vi "测量值存进数据库练习.vi"() -> ()   [LabVIEW 2025]
uses:
  <vilib>/Instr/_visa.llb/VISA Configure Serial Port (Instr).vi
panel:
  out "转换为十进制数据":u32
  out "地址01的光亮度数据":dbl
  out "字符串显示·的十六进制数据":string
  out "无符号字节数组":u8[](array[numeric])
  out "十六进制整形字符串":string[](array[string])
  out "提取的从机地址01的亮度原始数据":string
  out "所有测量记录":string[][](table)
  out "获取下位机返回的原始数据包":string
  in  "发送命令":string
  in  "波特率":u32=9600 caption="波特率(9600)"
  in  "选择串口":refnum<visa-resource-name>
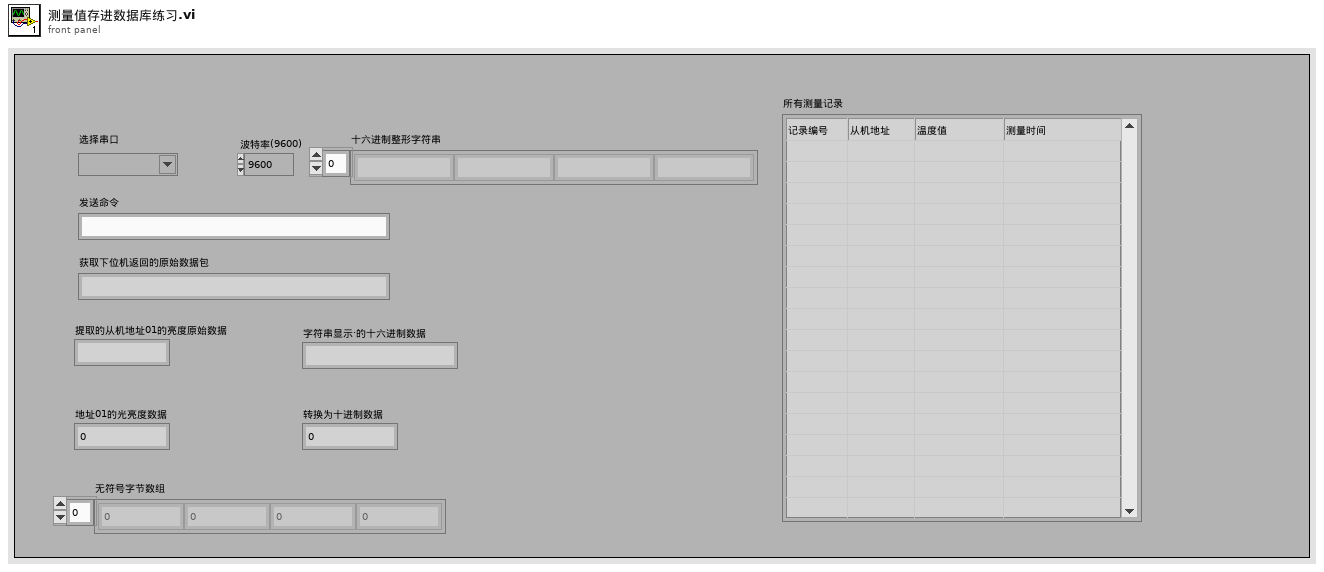
[diagram p1: front panel]
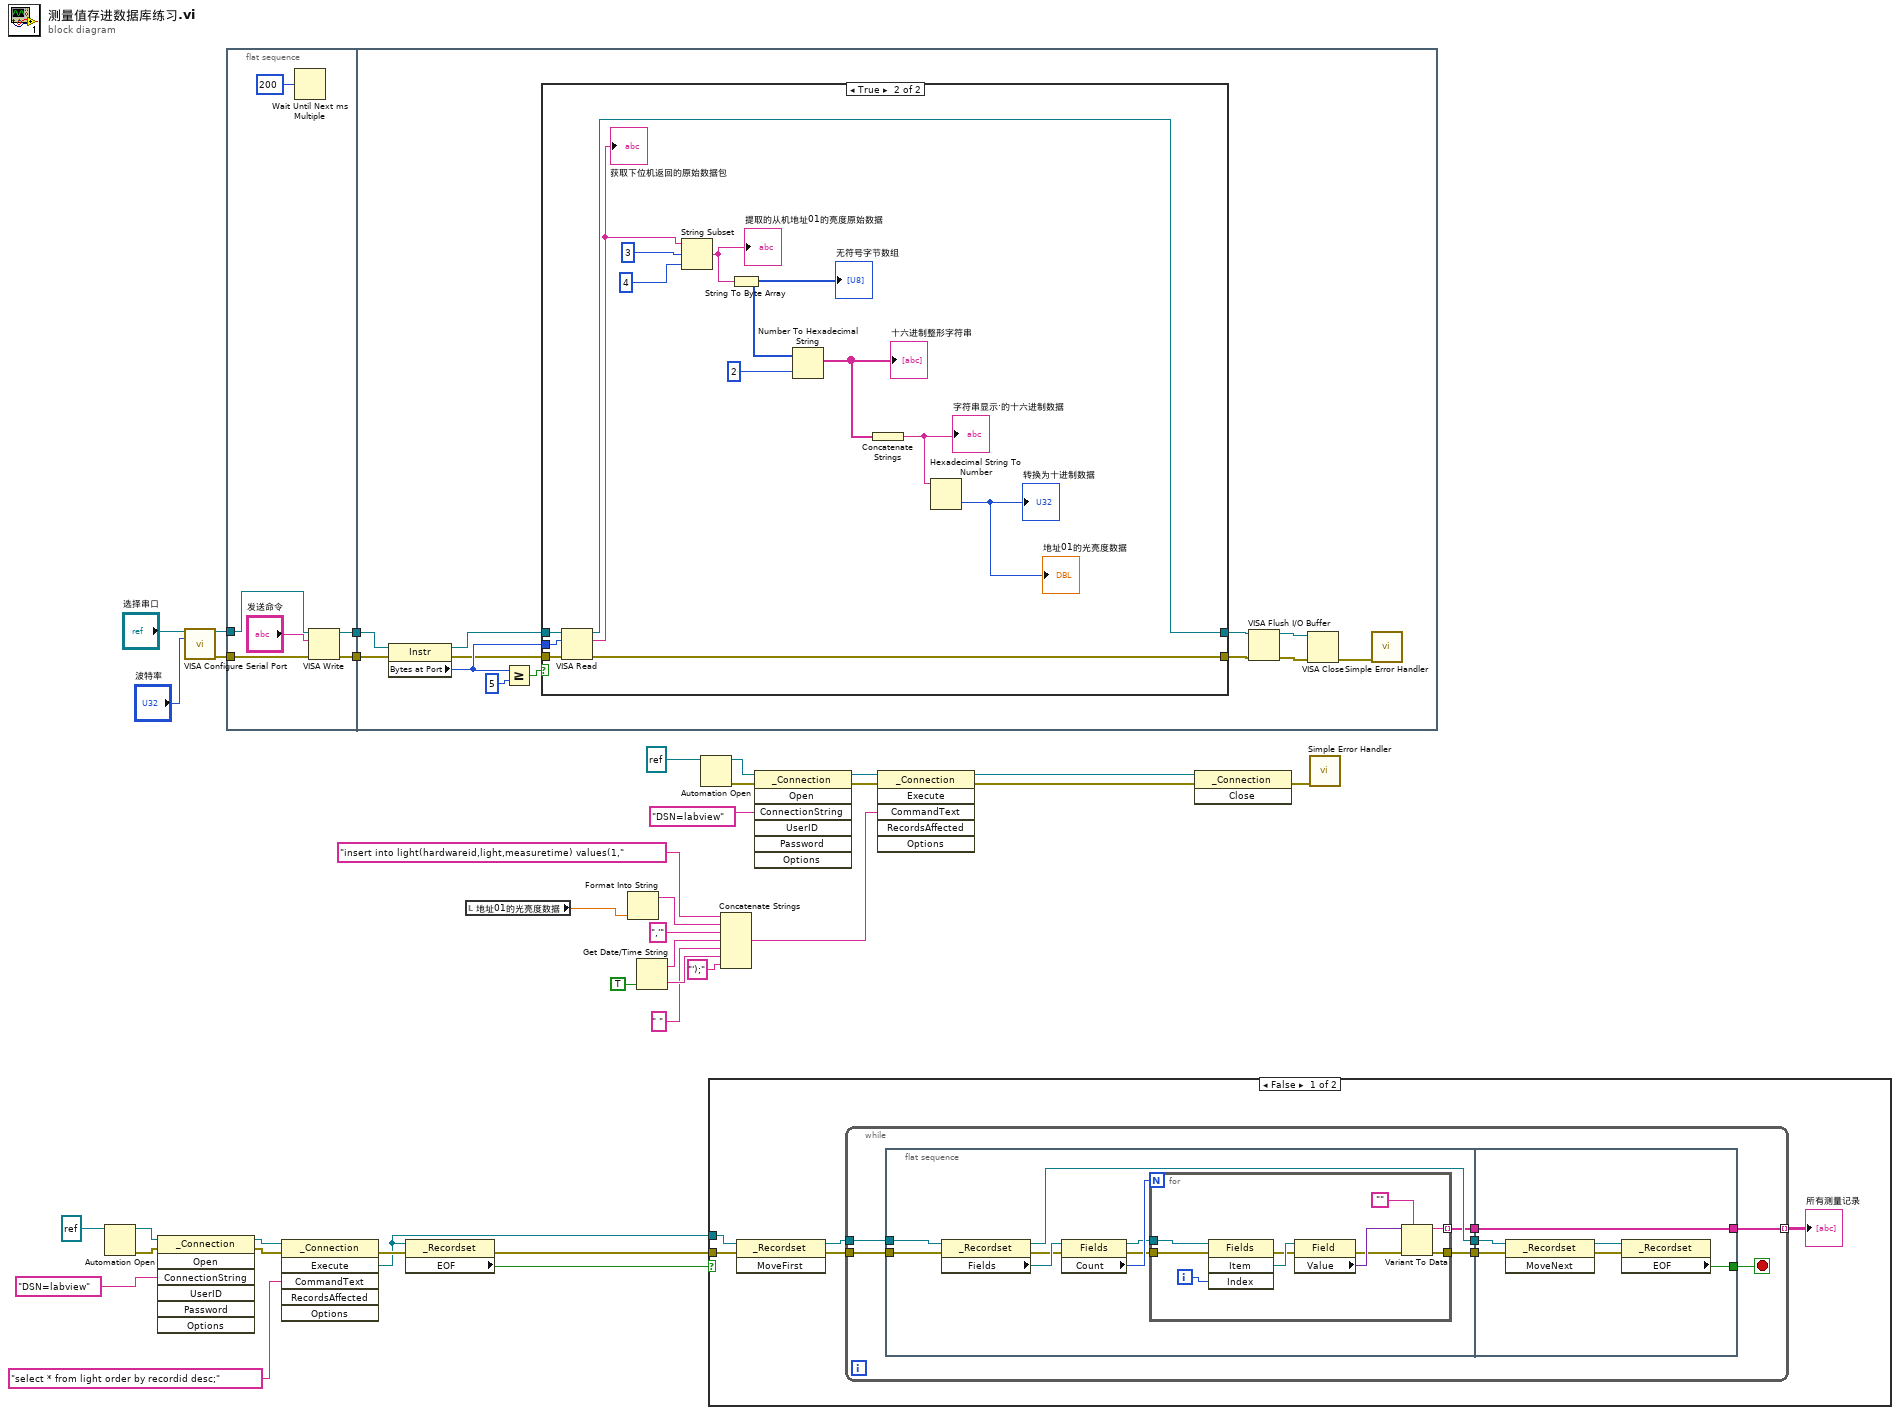
[diagram p0: block diagram]
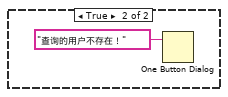
[diagram p2: hidden frame]
diagram:
  n1 = Automation Open(Automation Refnum=refnum<k7> refnum ("ADODB._Connection")) -> (Automation Refnum=w4:refnum<k7>, error out=w3:errorcluster)  [unwired: 3 in]
  n2 = invoke on="调用节点" class="_Connection" method="Open"(reference=w4, error in=w3, "ConnectionString"="DSN=labview") -> (reference out=w6:refnum<k7>, error out=w5:errorcluster)  [unwired: 4 in, 5 out]
  n3 = call-poly "VISA Configure Serial Port"("VISA resource name"="选择串口", "baud rate (9600)"="波特率") -> ("VISA resource name out"=w34:refnum<visa-resource-name>, "error out"=w33:errorcluster)  [unwired: 12 in]
  n4 = flat-sequence {
    tunnel: w34 -> [w41]
    tunnel: w33 -> [w40]
    tunnel: [w38] -> w32
    tunnel: [w37] -> w31
    tunnel: w32 -> [w54]
    tunnel: w31 -> [w53]
    frame #0 {
      n5 = Wait Until Next ms Multiple(millisecond multiple=u32 200 ("毫秒倍数")) -> ()  [unwired: 1 out]
      n6 = VISA Write(VISA resource name=w41, write buffer="发送命令", error in (no error)=w40) -> (VISA resource name out=w38:refnum<visa-resource-name>, error out=w37:errorcluster)  [unwired: 1 out]
    }
    frame #1 {
      n7 = property class="Instr"(reference=w54, error in=w53) -> (reference out=w50:refnum<visa-resource-name>, error out=w48:errorcluster, "Bytes at Port"=w49:u32)
      n8 = Greater Or Equal?(x=w49, y=u32 5) -> (x >= y?=w52:bool)
      n9 = case shown="True" w52 {
        tunnel: w50 -> [w56 w70]
        tunnel: w49 -> [_ w69]
        tunnel: w48 -> [w55 w68]
        tunnel: [w56 w67] -> w44
        tunnel: [w55 w66] -> w43
        frame False {
        }
        frame True {
          n10 = VISA Read(VISA resource name=w70, byte count=w69, error in (no error)=w68) -> (VISA resource name out=w67:refnum<visa-resource-name>, read buffer=w57:string, error out=w66:errorcluster)  [unwired: 1 out]
          "获取下位机返回的原始数据包" <- w57
          n11 = String Subset(string=w57, offset (0)=3 ("偏移量(0)"), length (rest)=4 ("长度（剩余）")) -> (substring=w63:string)
          "提取的从机地址01的亮度原始数据" <- w63
          n12 = String To Byte Array(string=w63) -> (unsigned byte array=w61:u8[])
          "无符号字节数组" <- w61
          n13 = Number To Hexadecimal String(1:i16 2 ("宽度(-)"), 2:w61) -> (0:w60:string[])
          "十六进制整形字符串" <- w60
          n14 = Concatenate Strings(w60) -> (w59:string)
          "字符串显示·的十六进制数据" <- w59
          n15 = Hexadecimal String To Number(string=w59) -> (number=→"地址01的光亮度数据" →"转换为十进制数据":u32)  [unwired: 2 in, 1 out]
        }
      }
      n16 = VISA Flush I/O Buffer(VISA resource name=w44, error in (no error)=w43) -> (VISA resource name out=w45:refnum<visa-resource-name>, error out=w46:errorcluster)  [unwired: 1 in]
      n17 = VISA Close(VISA resource name=w45, error in (no error)=w46) -> (error out=w47:errorcluster)
      n18 = call <vilib>:"Simple Error Handler.vi"("error in (no error)"=w47) -> ()  [unwired: 4 in, 5 out]
    }
  }
  n19 = invoke class="_Connection" method="Execute"(reference=w6, error in=w5, "CommandText"="select * from light order by recordid desc;") -> (error out=w28:errorcluster, "Execute"=w26:refnum<k7>)  [unwired: 3 in, 4 out]
  n20 = property class="_Recordset"(reference=w26, error in=w28) -> (error out=w25:errorcluster, "EOF"=w27:bool)  [unwired: 1 out]
  n21 = local read "地址01的光亮度数据"() -> (w1:dbl)
  n22 = Format Into String(w1) -> (resulting string=w24:string)  [unwired: 3 in, 1 out]
  n23 = Get Date/Time String(want seconds? (F)=TRUE) -> (date string=w17:string, time string=w18:string)  [unwired: 2 in]
  n24 = Automation Open(Automation Refnum=refnum<k7> refnum ("ADODB._Connection")) -> (Automation Refnum=w23:refnum<k7>, error out=w22:errorcluster)  [unwired: 3 in]
  n25 = case shown="False" w27 {
    tunnel: w26 -> [w75 _]
    tunnel: w25 -> [w74 _]
    frame False {
      n26 = invoke class="_Recordset" method="MoveFirst"(reference=w75, error in=w74) -> (reference out=w72:refnum<k7>, error out=w73:errorcluster)  [unwired: 1 in, 1 out]
      n27 = while {
        tunnel: w73 -> [w80]
        tunnel: w72 -> [w79]
        tunnel: [w76] -> w71 mode=indexing
        stop <- w78 stop-if-true
        n28 = flat-sequence {
          tunnel: w79 -> [w92]
          tunnel: w80 -> [w91]
          tunnel: [w85] -> w82
          tunnel: [w84] -> w81
          tunnel: [w83] -> w77
          tunnel: w82 -> [w106]
          tunnel: w81 -> [w105]
          tunnel: [w104] -> w78
          tunnel: w77 -> [w103]
          tunnel: [w103] -> w76
          frame #0 {
            n29 = property class="_Recordset"(reference=w92, error in=w91) -> (reference out=w84:refnum<k7>, error out=w89:errorcluster, "Fields"=w90:refnum<k7>)
            n30 = property class="Fields"(reference=w90, error in=w89) -> (reference out=w87:refnum<k7>, error out=w86:errorcluster, "Count"=w88:i32)
            n31 = for {
              N: w88 -> [_]
              tunnel: w87 -> [w97]
              tunnel: w86 -> [w96]
              tunnel: [w94] -> w83 mode=indexing
              tunnel: [w93] -> w85
              i -> [w95]
              n32 = invoke class="Fields" method="Item"(reference=w97, error in=w96, "Index"=w95) -> (error out=w101:errorcluster, "Item"=w102:refnum<k7>)  [unwired: 1 in, 2 out]
              n33 = property class="Field"(reference=w102, error in=w101) -> (error out=w98:errorcluster, "Value"=w99:variant)  [unwired: 1 out]
              n34 = Variant To Data(error in=w98, type="", Variant=w99) -> (data=w94:string, error out=w93:errorcluster)
            }
          }
          frame #1 {
            n35 = invoke class="_Recordset" method="MoveNext"(reference=w105, error in=w106) -> (reference out=w108:refnum<k7>, error out=w107:errorcluster)  [unwired: 1 in, 1 out]
            n36 = property class="_Recordset"(reference=w108, error in=w107) -> ("EOF"=w104:bool)  [unwired: 2 out]
          }
        }
      }
      "所有测量记录" <- w71
    }
    frame True {
      n37 = One Button Dialog(message="查询的用户不存在！") -> ()  [unwired: 1 in, 1 out]
    }
  }
  n38 = Concatenate Strings("insert into light(hardwareid,light,measuretime) values(1," ("CommandText"), w24, ",'" ("字符串"), w17, " " ("string"), w18, "');" ("string")) -> (w19:string)
  n39 = invoke class="_Connection" method="Open"(reference=w23, error in=w22, "ConnectionString"="DSN=labview") -> (reference out=w21:refnum<k7>, error out=w20:errorcluster)  [unwired: 4 in, 5 out]
  n40 = invoke class="_Connection" method="Execute"(reference=w21, error in=w20, "CommandText"=w19) -> (reference out=w8:refnum<k7>, error out=w7:errorcluster)  [unwired: 3 in, 4 out]
  n41 = invoke class="_Connection" method="Close"(reference=w8, error in=w7) -> (error out=w9:errorcluster)  [unwired: 1 in, 2 out]
  n42 = call <vilib>:"Simple Error Handler.vi"("error in (no error)"=w9) -> ()  [unwired: 4 in, 5 out]
